vi "getName.vi"(8 "error in (no error)":errorcluster, 11 "bike in":refnum<class "bike.lvclass">) -> (0 "error out":errorcluster, 2 "name":string, 3 "bike out":refnum<class "bike.lvclass">)   [LabVIEW 2011, in "bike.lvclass"]
uses:
  bike.lvclass
  genericVehicle/vehicleGeneric.lvclass
  bike.lvclass/bike.ctl
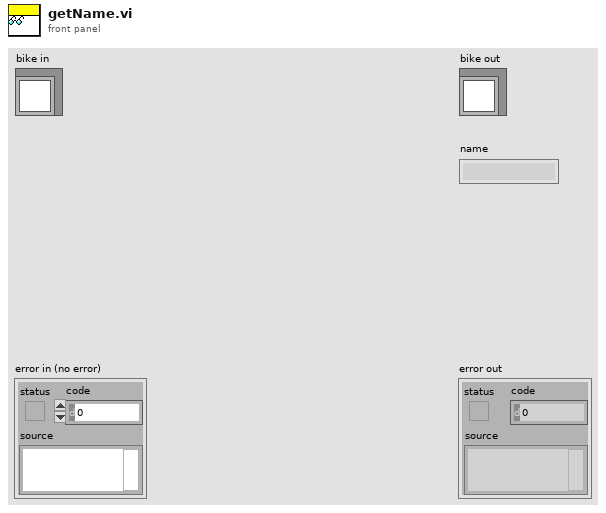
[diagram p1: front panel]
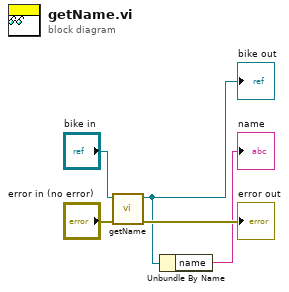
[diagram p0: block diagram]
diagram:
  n1 = call-parent "getName.vi"("error in (no error)"="error in (no error)", "vehicleGeneric in"="bike in") -> ("error out"=→"error out":errorcluster, "vehicleGeneric out"=w2:refnum<class "bike.lvclass">)  [unwired: 7 in, 1 out]
  "bike out" <- w2
  n2 = Unbundle By Name(w2) -> ("name"=→"name":string)
